vi "Init.vi"(8 "error in (no error)":errorcluster, 11 "config in":T1) -> (0 "error out":errorcluster, 3 "config out":T1)   [LabVIEW 2017, in "EmsaAudio.lvlib"]
uses:
  <vilib>/addons/InsightCM/Devices/Shared/Emsa/EmsaAudio/EmsaAudio.lvlib
  <vilib>/addons/InsightCM/Devices/Shared/Emsa/EmsaAudio/controls/config.ctl
  <vilib>/addons/InsightCM/Utilities/GlobalConfiguration/GlobalConfiguration.lvlib
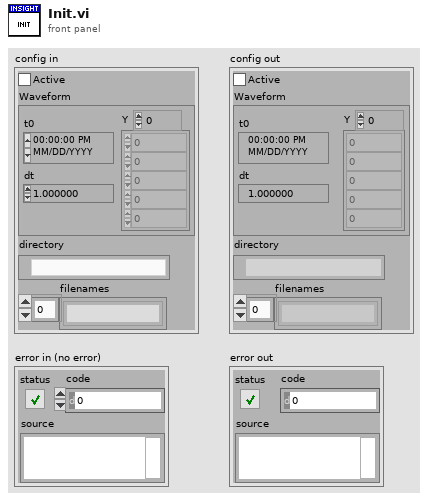
[diagram p1: front panel]
types:
  T1 = typedef "EmsaAudio.lvlib/config.ctl" = cluster{"Active":bool, "Waveform":waveform(dbl), "directory":path, "filenames":string[]}
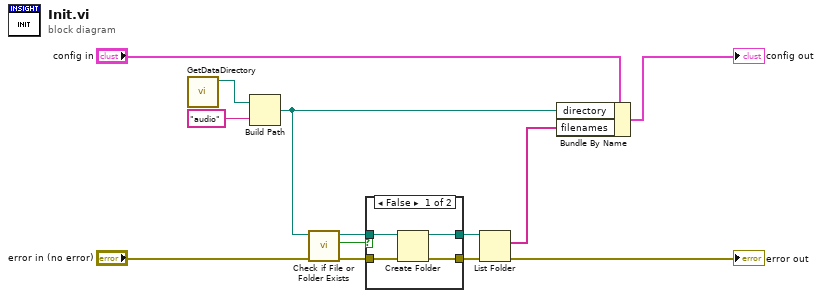
[diagram p0: block diagram]
diagram:
  n1 = call <vilib>:"GetDataDirectory.vi"() -> ("data directory"=w13:path)  [unwired: 10 in, 1 out]
  n2 = Build Path(base path=w13, name or relative path="audio") -> (appended path=w9:path)
  n3 = call <vilib>:"Check if File or Folder Exists.vi"("error in (no error)"="error in (no error)", "path"=w9) -> ("error out"=w5:errorcluster, "file or folder exists?"=w4:bool, "dup path"=w3:path)  [unwired: 7 in]
  n4 = case shown="False" w4 {
    tunnel: w5 -> [w16 w19]
    tunnel: [w14 w19] -> w7
    tunnel: w3 -> [w17 w18]
    tunnel: [w15 w18] -> w6
    frame False {
      n5 = Create Folder(path (use dialog)=w17, error in=w16) -> (created path=w15:path, error out=w14:errorcluster)  [unwired: 1 in, 1 out]
    }
    frame True {
    }
  }
  n6 = List Folder(path=w6, error in=w7) -> (filenames=w11:string[], error out=→"error out":errorcluster)  [unwired: 2 in, 2 out]
  n7 = Bundle By Name(cluster="config in", "directory"=w9, "filenames"=w11) -> (→"config out":T1)
